vi "BLE_DataAquisition.vi"() -> ()   [LabVIEW 2020]
uses:
  BLE_Data.ctl
  BLE_Message.ctl
  BLE_Message_Info.ctl
  BLE_Response.ctl
  BLE_Response_Info.ctl
  Main_Data.ctl
  C:/Users/Trait/Repos/BLE_BeaconSensor/BLE_ClientPC/BLELib.dll
  BLELib.dll
  BLE.lvlib
panel:
  out "Discovered devices":string[](array[string])
  out "BLE Loop":bool
  out "Main Loop":bool
  in  "Start_aquisition_btn":bool
  out "Device_found_led":bool
  in  "Scan_btn":bool
  in  "Stop_btn":bool
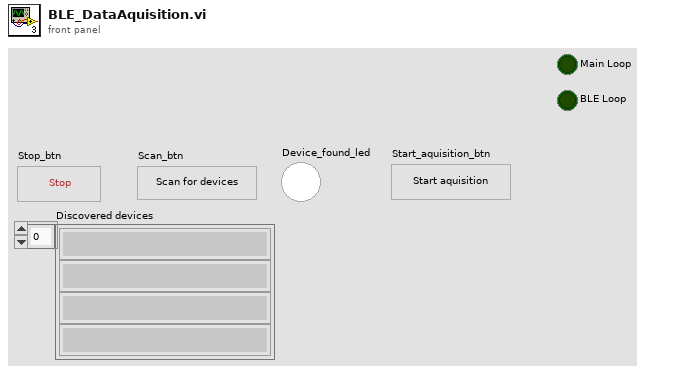
[diagram p1: front panel]
types:
  T1 = typedef "Main_Data.ctl" = cluster{"Scanned Devices":string[]}
  T2 = typedef "BLE_Response.ctl" = cluster{"BLE_Info":T3, "BLE_Data":variant}
  T3 = typedef "BLE_Response_Info.ctl" = enum16{"ScannedDevices"}
  T4 = typedef "BLE_Message.ctl" = cluster{"BLE_Parameter":variant, "BLE_Command":T5}
  T5 = typedef "BLE_Message_Info.ctl" = enum16{"Idle", "Init", "ScanToogle", "Connect", "Exit"}
  T6 = typedef "BLE_Data.ctl" = cluster{".NET Ref":refnum<k24>, "IsScanning?":bool}
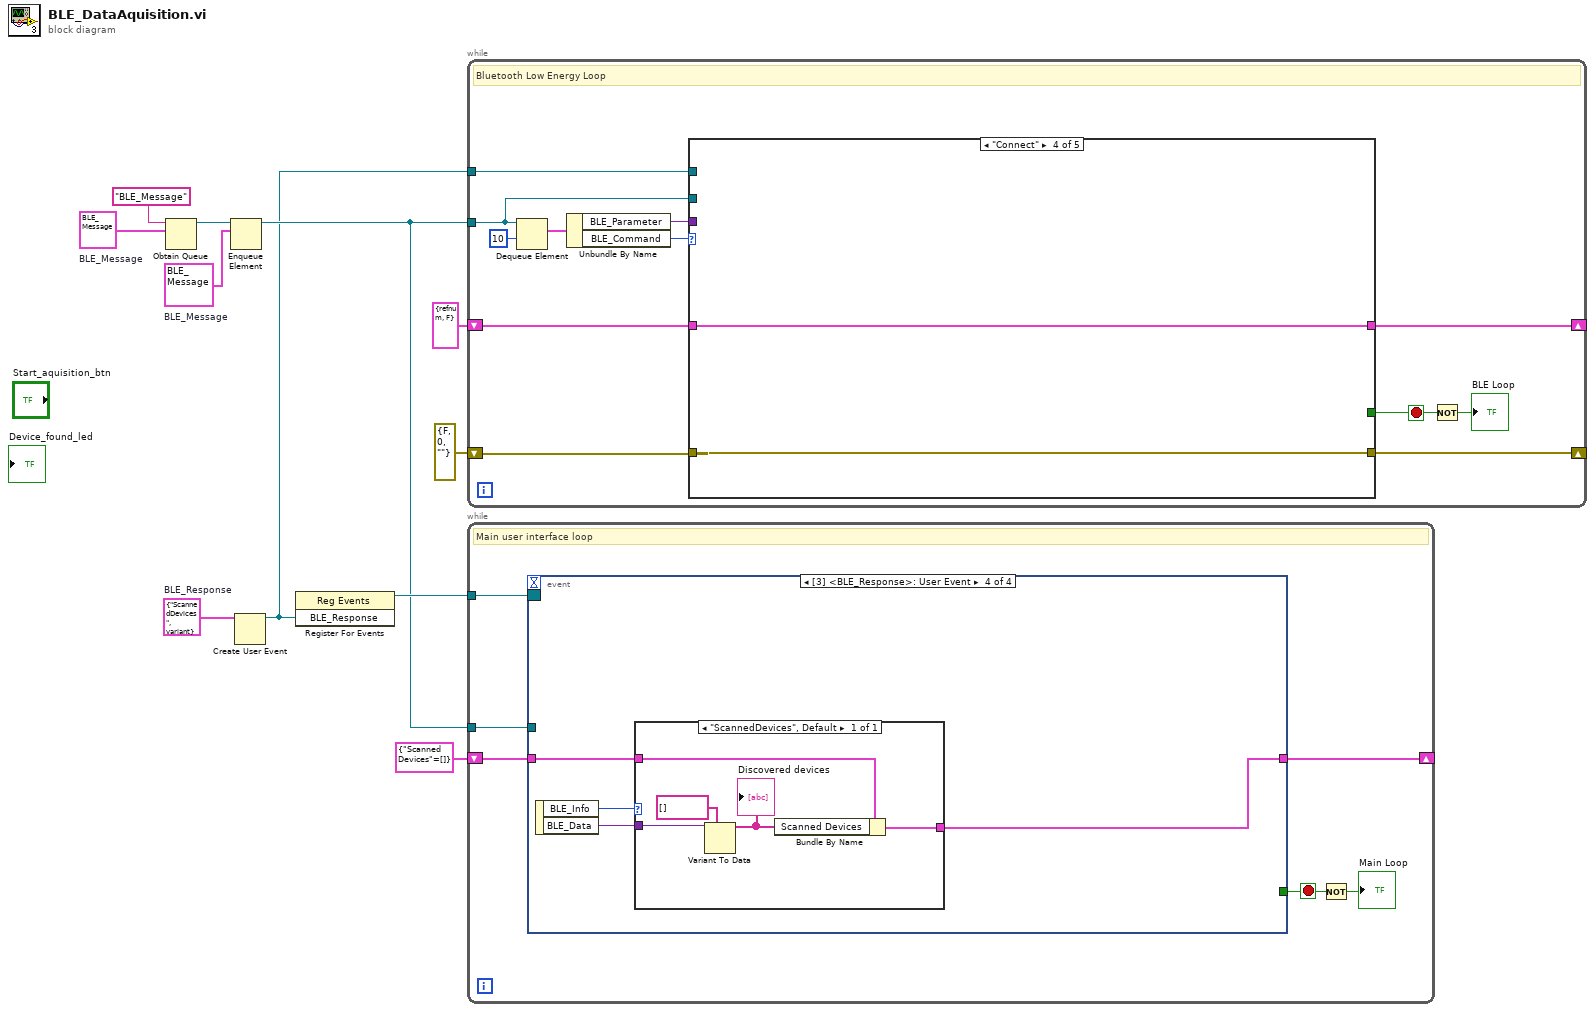
[diagram p0: block diagram]
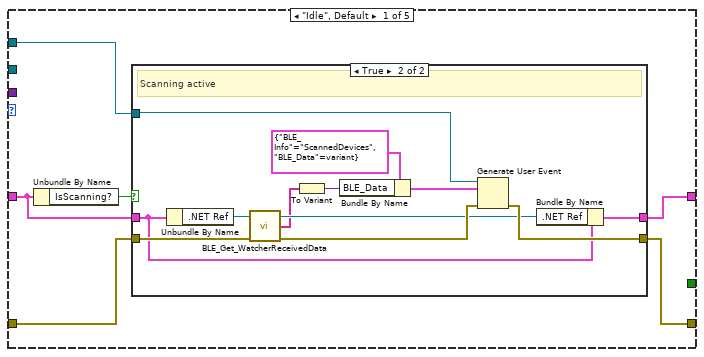
[diagram p2: hidden frame]
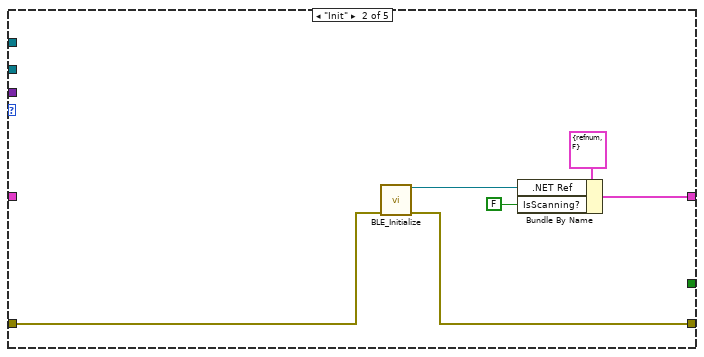
[diagram p4: hidden frame]
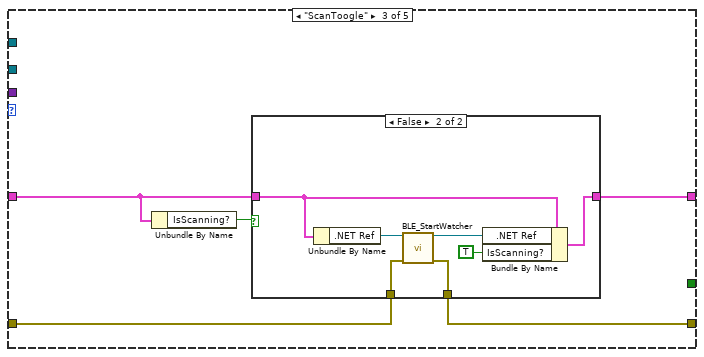
[diagram p5: hidden frame]
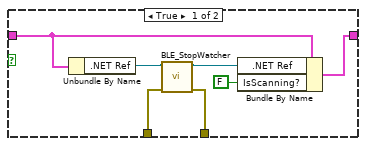
[diagram p6: hidden frame]
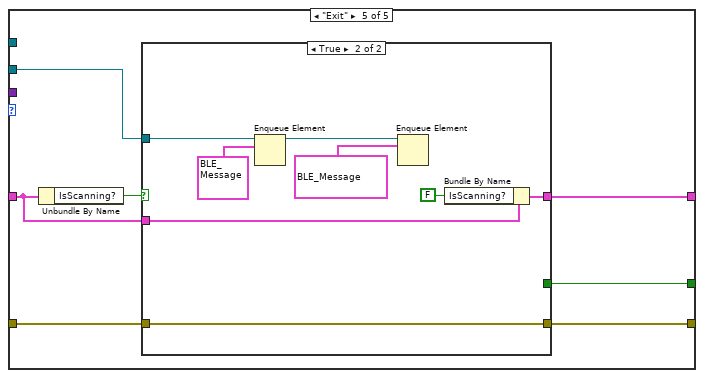
[diagram p7: hidden frame]
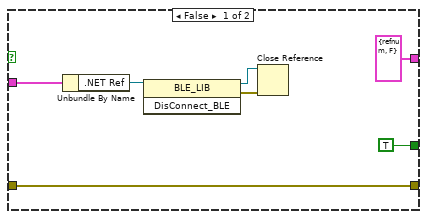
[diagram p8: hidden frame]
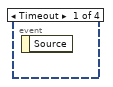
[diagram p9: hidden frame]
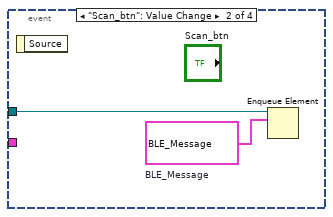
[diagram p10: hidden frame]
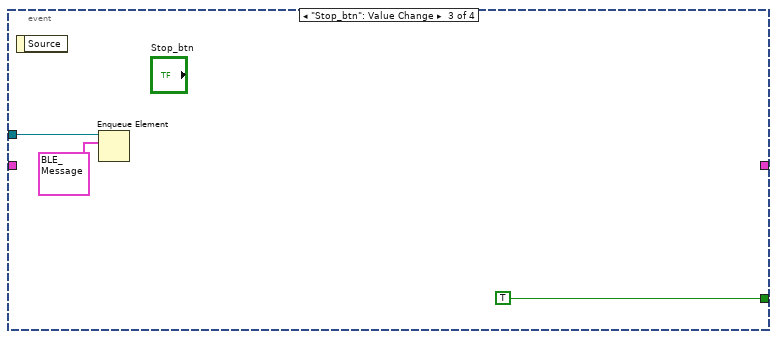
[diagram p11: hidden frame]
diagram:
  w3 = T2 {"BLE_Info"=enum."ScannedDevices", "BLE_Data"=variant}  # BLE_Response
  w4 = T4 {"BLE_Parameter"=variant, "BLE_Command"=enum."Init"}  # BLE_Message
  w8 = T4 {"BLE_Parameter"=variant, "BLE_Command"=enum."Idle"}  # BLE_Message
  n1 = Obtain Queue(name (unnamed)="BLE_Message", element data type=w8) -> (queue out=w6:refnum<queue>)  [unwired: 3 in, 2 out]
  n2 = Enqueue Element(queue=w6, element=w4) -> (queue out=w5:refnum<queue>)  [unwired: 2 in, 2 out]
  n3 = Create User Event(user event datatype=w3) -> (user event=w2:refnum<user-event>)  [unwired: 1 in, 1 out]
  n4 = register-events(w2) -> (reference out=w7:refnum<event-registration>)  [unwired: 2 in, 1 out]
  n5 = while {
    shift-right: [w21] -> _
    shift-left: T6 {".NET Ref"=refnum, "IsScanning?"=FALSE} -> [w17]
    shift-right: [w23] -> _
    shift-left: errorcluster {"status"=FALSE, "code"=0, "source"=""} ("error constant") -> [w22]
    tunnel: w5 -> [w14]
    tunnel: w2 -> [w15]
    stop <- w13 stop-if-true
    # "Bluetooth Low Energy Loop"
    n6 = Dequeue Element(queue=w14, timeout in ms (-1)=10) -> (element=w19:T4)  [unwired: 1 in, 3 out]
    n7 = Unbundle By Name(w19) -> ("BLE_Parameter"=w16:variant, "BLE_Command"=w18:T5)
    n8 = case shown="\"Connect\"" w18 {
      tunnel: w22 -> [w28 w49 w54 w69 w73]
      tunnel: [w27 w48 w53 w69 w72] -> w23
      tunnel: [w24 w44 w52 w70 w75] -> w21
      tunnel: w17 -> [w25 _ w51 w70 w74]
      tunnel: w16 -> [_ _ _ _ _]
      tunnel: w15 -> [w26 _ _ _ _]
      tunnel: w14 -> [_ _ _ _ w76]
      tunnel: [_ _ _ _ w71] -> w13
      frame "Idle", Default {
        n9 = Unbundle By Name(w25) -> ("IsScanning?"=w29:bool)
        n10 = case shown="True" w29 {
          tunnel: w28 -> [w31 w43]
          tunnel: [w31 w41] -> w27
          tunnel: w26 -> [_ w35]
          tunnel: w25 -> [w30 w37]
          tunnel: [w30 w36] -> w24
          frame False {
            # "Scanning not active"
          }
          frame True {
            # "Scanning active"
            n11 = Unbundle By Name(w37) -> (".NET Ref"=w39:refnum<k24>)
            n12 = call "BLE_Get_WatcherReceivedData.vi"(".NET Refnum in"=w39, "error in (no error)"=w43) -> (".NET Refnum out"=w38:refnum<k24>, "Bluetooth Addr"=w32:string[], "error out"=w42:errorcluster)  [unwired: 6 in, 5 out]
            n13 = To Variant(anything=w32) -> (Variant=w40:variant)
            n14 = Bundle By Name(cluster=T2 {"BLE_Info"=enum."ScannedDevices", "BLE_Data"=variant}, "BLE_Data"=w40) -> (w33:T2)
            n15 = Generate User Event(user event=w35, event data cluster=w33, error in=w42) -> (error out=w41:errorcluster)  [unwired: 1 in, 1 out]
            n16 = Bundle By Name(cluster=w37, ".NET Ref"=w38) -> (w36:T6)
          }
        }
      }
      frame "Init" {
        n17 = call "BLE_Initialize.vi"("error in (no error)"=w49) -> (".NET Refnum out"=w46:refnum<k24>, "error out"=w48:errorcluster)  [unwired: 13 in]
        n18 = Bundle By Name(cluster=T6 {".NET Ref"=refnum, "IsScanning?"=FALSE}, ".NET Ref"=w46, "IsScanning?"=FALSE) -> (w44:T6)
      }
      frame "ScanToogle" {
        n19 = Unbundle By Name(w51) -> ("IsScanning?"=w50:bool)
        n20 = case shown="False" w50 {
          tunnel: w54 -> [w56 w68]
          tunnel: [w55 w67] -> w53
          tunnel: w51 -> [w57 w63]
          tunnel: [w58 w62] -> w52
          frame True {
            n21 = Unbundle By Name(w57) -> (".NET Ref"=w61:refnum<k24>)
            n22 = call "BLE_StopWatcher.vi"(".NET Refnum in"=w61, "error in (no error)"=w56) -> (".NET Refnum out"=w60:refnum<k24>, "error out"=w55:errorcluster)  [unwired: 11 in, 1 out]
            n23 = Bundle By Name(cluster=w57, ".NET Ref"=w60, "IsScanning?"=FALSE) -> (w58:T6)
          }
          frame False {
            n24 = Unbundle By Name(w63) -> (".NET Ref"=w64:refnum<k24>)
            n25 = call "BLE_StartWatcher.vi"(".NET Refnum in"=w64, "error in (no error)"=w68) -> (".NET Refnum out"=w66:refnum<k24>, "error out"=w67:errorcluster)  [unwired: 11 in, 1 out]
            n26 = Bundle By Name(cluster=w63, ".NET Ref"=w66, "IsScanning?"=TRUE) -> (w62:T6)
          }
        }
      }
      frame "Connect" {
      }
      frame "Exit" {
        n27 = Unbundle By Name(w74) -> ("IsScanning?"=w77:bool)
        n28 = case shown="True" w77 {
          tunnel: w76 -> [_ w92]
          tunnel: [T6 {".NET Ref"=refnum, "IsScanning?"=FALSE} w89] -> w75
          tunnel: w74 -> [w83 w88]
          tunnel: w73 -> [w84 w86]
          tunnel: [w84 w86] -> w72
          tunnel: [TRUE _] -> w71
          frame False {
            n29 = Unbundle By Name(w83) -> (".NET Ref"=w80:refnum<k24>)
            n30 = invoke class="BLE_LIB" method="DisConnect_BLE"(reference=w80) -> (reference out=w82:refnum<k24>, error out=w81:errorcluster)  [unwired: 2 in, 1 out]
            n31 = Close Reference(reference=w82, error in (no error)=w81) -> ()  [unwired: 1 out]
          }
          frame True {
            n32 = Enqueue Element(queue=w92, element=T4 {"BLE_Parameter"=variant, "BLE_Command"=enum."Exit"}) -> (queue out=w91:refnum<queue>)  [unwired: 2 in, 2 out]
            n33 = Enqueue Element(queue=w91, element=T4 {"BLE_Parameter"=variant, "BLE_Command"=enum."ScanToogle"}) -> ()  [unwired: 2 in, 3 out]
            n34 = Bundle By Name(cluster=w88, "IsScanning?"=FALSE) -> (w89:T6)
          }
        }
      }
    }
    n35 = Not(x=w13) -> (.not. x?=→"BLE Loop":bool)
  }
  n36 = while {
    tunnel: w5 -> [w97]
    tunnel: w7 -> [w96]
    shift-right: [w94] -> _
    shift-left: T1 {"Scanned Devices"=[]} -> [w93]
    stop <- w98 stop-if-true
    # "Main user interface loop"
    n37 = event shown="[3] <BLE_Response>: User Event" {
      selector: w96 -> [_ _ _ _]
      dyn-events: _ -> [_ _ _ _]
      timeout: _ -> [_ _ _ _]
      tunnel: [_ _ TRUE _] -> w98
      tunnel: w97 -> [_ w100 w103 _]
      tunnel: [_ _ _ w105] -> w94
      tunnel: w93 -> [_ _ _ w104]
      event Timeout {
        n38 = event-data() -> ()  [unwired: 1 in, 1 out]
      }
      event "Scan_btn": Value Change {
        w99 = T4 {"BLE_Parameter"=variant, "BLE_Command"=enum."ScanToogle"}  # BLE_Message
        n39 = event-data() -> ()  [unwired: 1 in, 1 out]
        n40 = Enqueue Element(queue=w100, element=w99) -> ()  [unwired: 2 in, 3 out]
      }
      event "Stop_btn": Value Change {
        n41 = event-data() -> ()  [unwired: 1 in, 1 out]
        n42 = Enqueue Element(queue=w103, element=T4 {"BLE_Parameter"=variant, "BLE_Command"=enum."Exit"}) -> ()  [unwired: 2 in, 3 out]
      }
      event User Event {
        n43 = event-data() -> ("BLE_Info"=w107:T3, "BLE_Data"=w106:variant)  [unwired: 1 in]
        n44 = case shown="\"ScannedDevices\", Default" w107 {
          tunnel: w106 -> [w112]
          tunnel: [w109] -> w105
          tunnel: w104 -> [w108]
          frame "ScannedDevices", Default {
            n45 = Variant To Data(type=string[] [], Variant=w112) -> (data=w110:string[])  [unwired: 1 in, 1 out]
            "Discovered devices" <- w110
            n46 = Bundle By Name(cluster=w108, "Scanned Devices"=w110) -> (w109:T1)
          }
        }
      }
    }
    n47 = Not(x=w98) -> (.not. x?=→"Main Loop":bool)
  }
